vi "Speed_calc.vi"(10 "X":dbl, 11 "Y":dbl) -> (2 "Vy":dbl, 3 "Vx":dbl)   [LabVIEW 2017, in "myPAM.lvlib"]
uses:
  myPAM.lvlib
panel:
  out "V":dbl
  out "Speed_loop":i32
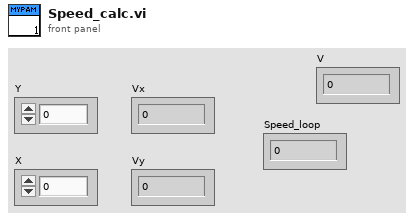
[diagram p1: front panel]
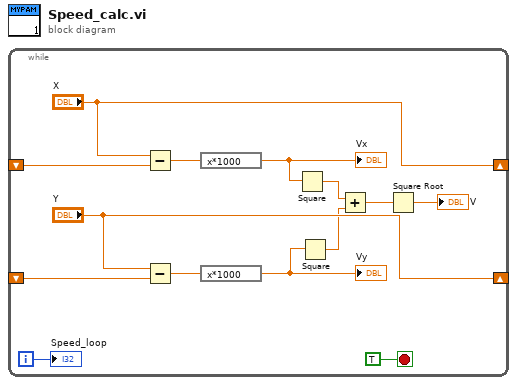
[diagram p0: block diagram]
diagram:
  n1 = while {
    shift-right: ["Y"] -> _
    shift-left: _ -> [w13]
    shift-right: ["X"] -> _
    shift-left: _ -> [w11]
    i -> [w7]
    stop <- TRUE stop-if-true
    n2 = Subtract(x="X", y=w11) -> (x-y=w9:dbl)
    n3 = Subtract(x="Y", y=w13) -> (x-y=w8:dbl)
    n4 = expression code="x*1000"(w9) -> (w5:dbl)
    "Vx" <- w5
    n5 = expression code="x*1000"(w8) -> (w6:dbl)
    "Vy" <- w6
    n6 = Square(x=w5) -> (x^2=w4:dbl)
    n7 = Square(x=w6) -> (x^2=w3:dbl)
    n8 = Add(x=w4, y=w3) -> (x+y=w2:dbl)
    n9 = Square Root(x=w2) -> (sqrt(x)=→"V":dbl)
    "Speed_loop" <- w7
  }
